vi "Esophogeal_HRME_Main.vi"() -> ()   [LabVIEW 2021]
uses:
  typeDefs/Esophogeal_Software_States.ctl
  <vilib>/DAQmx/read.llb/DAQmx Read (Digital 1D Bool NChan 1Samp 1Line).vi
  <extravilib>/ChannelInstances/High Speed Stream-str/_Read For Replicate.vi
  <extravilib>/ChannelInstances/High Speed Stream-a[.,.](u8)/_Read For Replicate.vi
  <vilib>/DAQmx/create/channels.llb/DAQmx Create Channel (DI-Digital Input).vi
  <vilib>/DAQmx/miscellaneous.llb/DAQmx Fill In Error Info.vi
  <extravilib>/ChannelInstances/High Speed Stream-str/Instantiate.vi
  <extravilib>/ChannelInstances/High Speed Stream-a[.,.](u8)/Instantiate.vi
  <extravilib>/ChannelInstances/High Speed Stream-str/)Channel.vi
  <extravilib>/ChannelInstances/High Speed Stream-str/Abort Signal/Init Signal.vi
  <extravilib>/ChannelInstances/High Speed Stream-a[.,.](u8)/)Channel.vi
  <extravilib>/ChannelInstances/High Speed Stream-a[.,.](u8)/Abort Signal/Init Signal.vi
  <vilib>/vision/driver/NI_Vision_Acquisition_Software.lvlib
  <resource>/objmgr/imaqdx.rc
  <extravilib>/ChannelInstances/High Speed Stream-a[.,.](u8).lvlib
  <extravilib>/ChannelInstances/High Speed Stream-str.lvlib
  <vilib>/vision/NI_Vision_Development_Module.lvlib
panel:
  out "Pause Status":bool
  in  "Tab Control":enum32{"Main Page", "Image Session Info"}(tab)
  in  "MTN Threshold:":enum16{"24.0", "15.9"}(ring)
  out "Image Analysis Meter":dbl(slide) scale=0.0..100.0
  in  "Calibrate":bool
  out "Saved Imaged Number":i32=1 caption="Number of Images Saved"
  out "Image Save Notification":string
  in  "Auto Gain":bool=TRUE
  in  "Auto Exposure":bool=TRUE
  in  "Save Button":bool
  out "Recording":bool
  in  "Play Button":bool
  in  "Close Program":bool
  in  "Pause Button":bool
  in  "HRME Gain":dbl(slide)=18.0 scale=0.0..30.0
  in  "HRME Exposure":dbl(slide)=7000.0 scale=100.0..80000.0
  out "HRME Image":T1(plugin-control)
  out "HRME Path":path
  out "HRME Scores":path
  out "Representative Images":path
  out "error out":errorcluster
  out "Patient Folder":path
  in  "Command File Location":path=path "C:/Users/EsophaHRME_Dell2/Documents/GitHub/Esophageal_HRME_Software/EsophagealDeployment/Multi_Task_Network/CommandFiles/LabVIEW/cmds.json"
  in  "Python Module Path":path=path "C:/Users/EsophaHRME_Dell2/Documents/GitHub/Esophageal_HRME_Software/EsophagealDeployment/Multi_Task_Network/mainv6.py"
  out "Log File Out":refnum<file>
  out "Anal HRME States":T2
  out "Timestamp":string
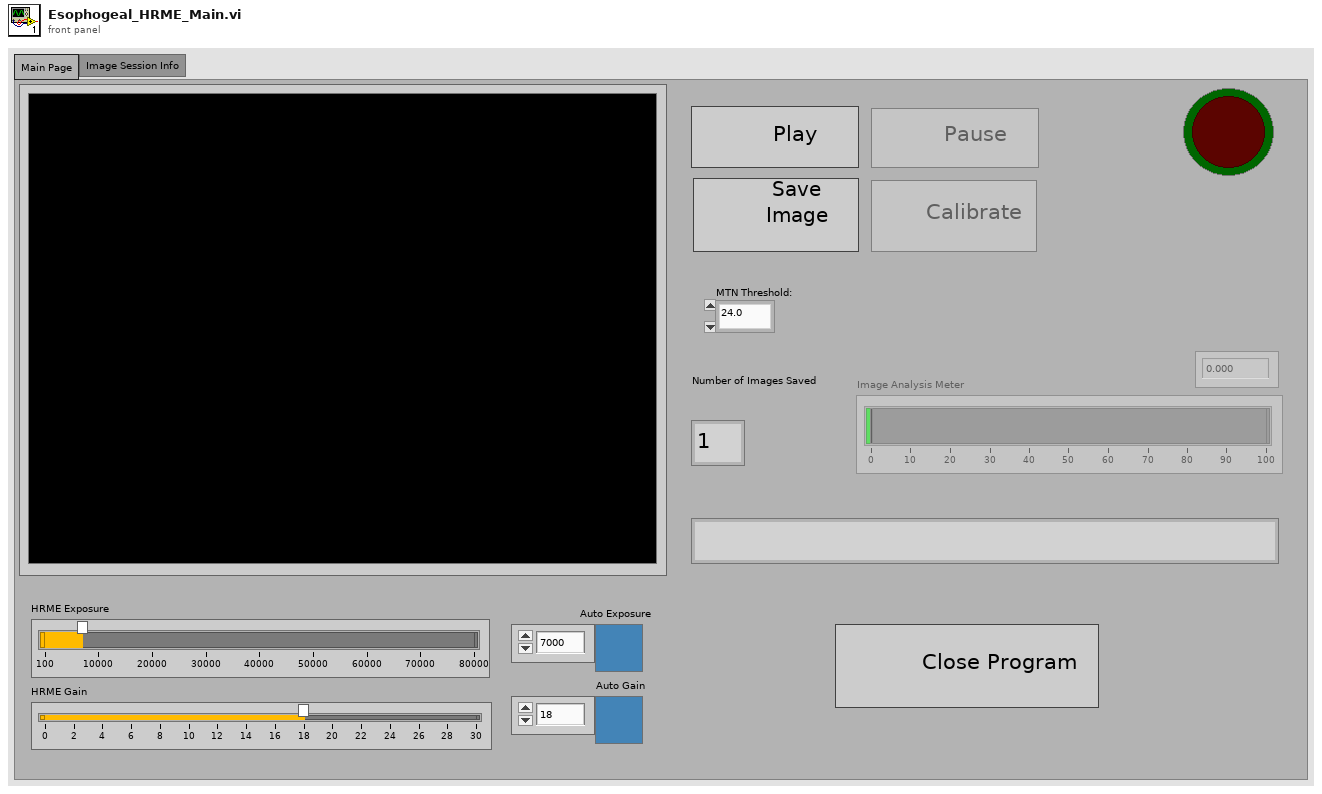
[diagram p1: front panel]
types:
  T1 = typedef "IMAQ Image.ctl" = refnum<image>
  T2 = typedef "Esophogeal_Software_States.ctl" = enum16{"Initialize", "Image Prep Screen", "Imaging", "Image Pause Screen", "Exit"}
  T3 = enum8{"Enabled", "Disabled", "Disabled and Grayed Out"}
  T4 = enum16{"open", "replace", "create", "open or create", "replace or create", "replace or create with confirmation"}
  T5 = cluster{"Source":string, "Destination":string, "CMD":string, "Time":string}
  T6 = typedef "IMAQdx.ctl" = refnum<k21>
  T7 = typedef "Image Type" = u32
  T8 = typedef "ROI Descriptor" = cluster{"Global Rectangle":i32[], "Contours":cluster{"ID":enum32{"External", "Internal"}, "Type":u32, "Coordinates":i32[]}[]}
  T9 = typedef "High Speed Stream-str.lvlib/)Channel.ctl" = refnum<queue>
  T10 = typedef "High Speed Stream-a[.,.](u8).lvlib/)Channel.ctl" = refnum<queue>
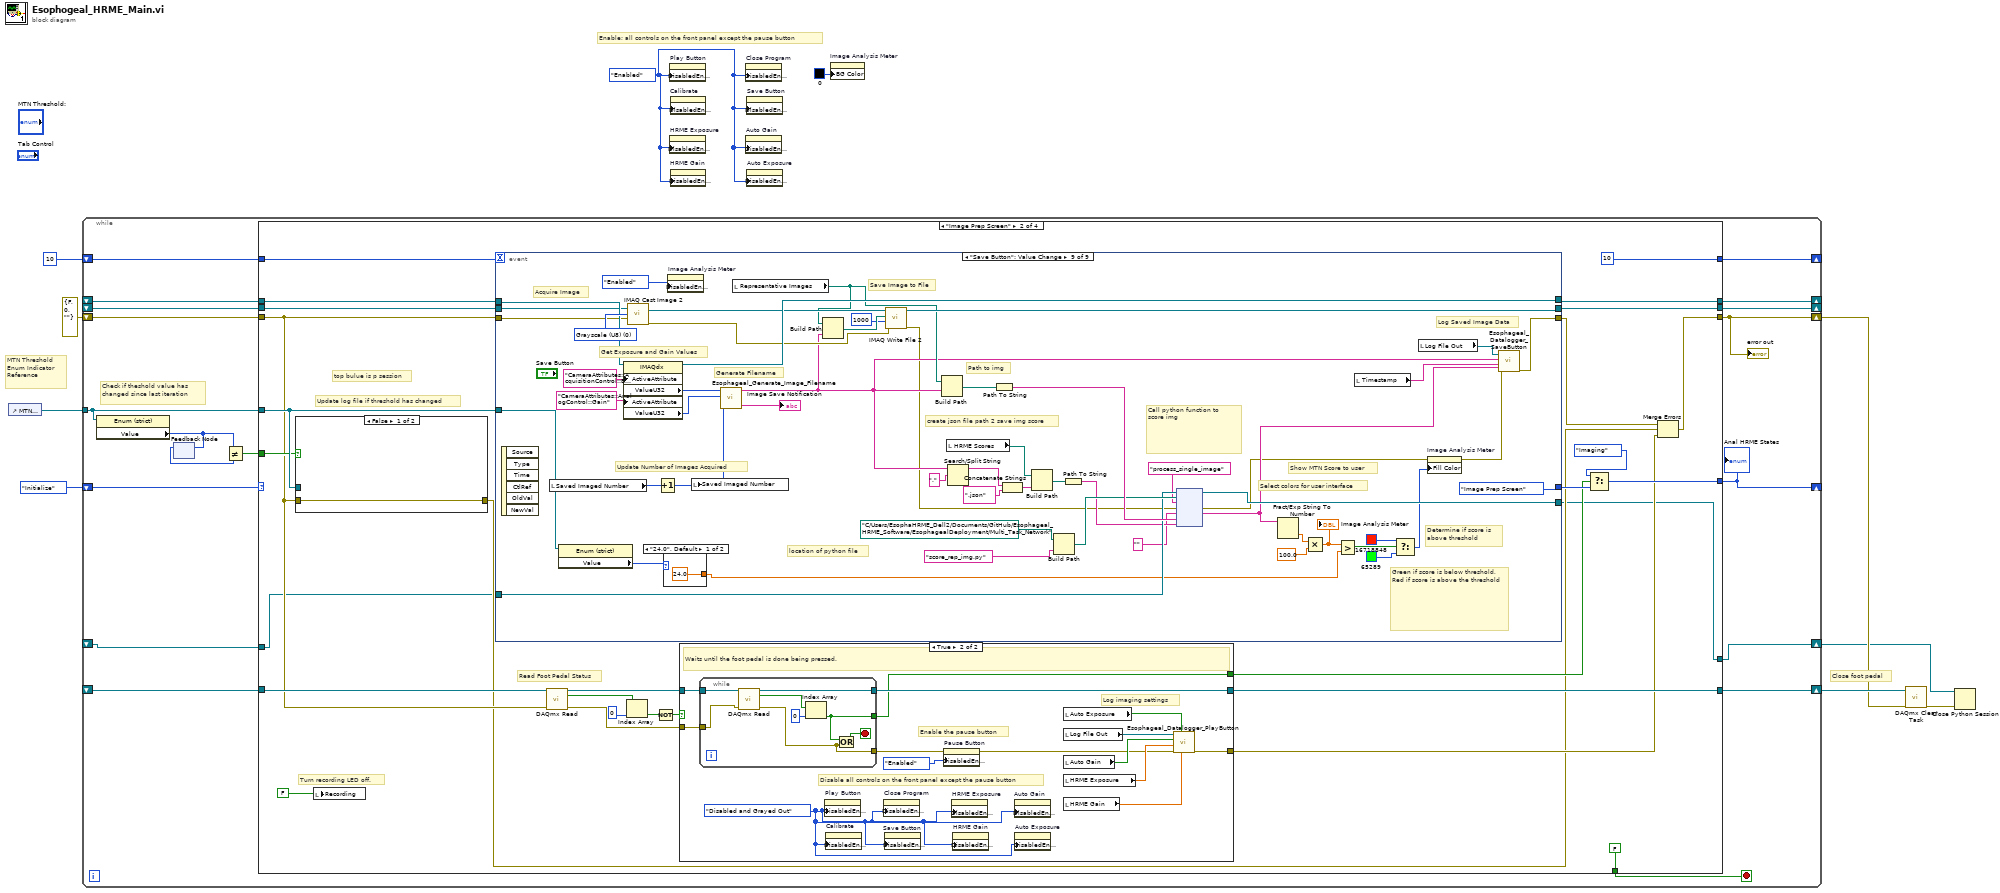
[diagram p0: block diagram]
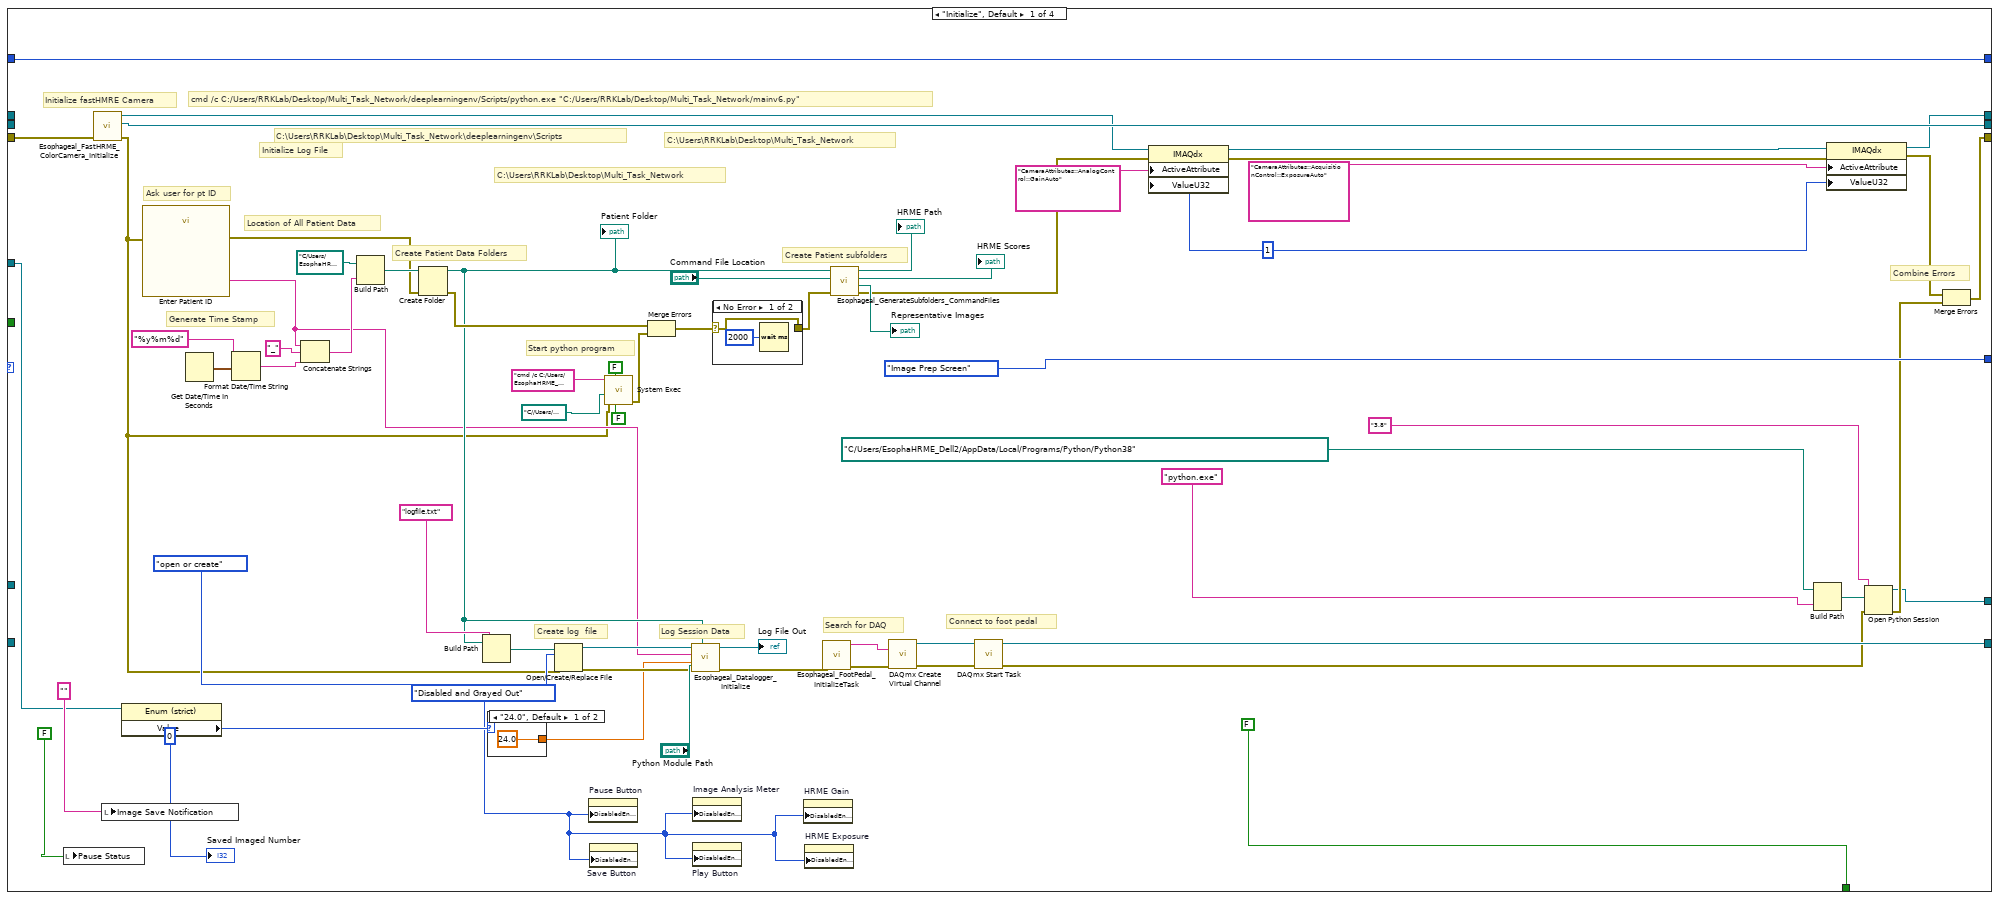
[diagram p2: hidden frame]
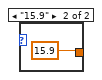
[diagram p3: hidden frame]
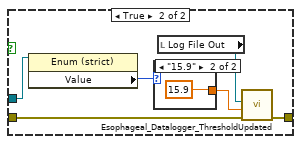
[diagram p5: hidden frame]
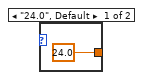
[diagram p6: hidden frame]
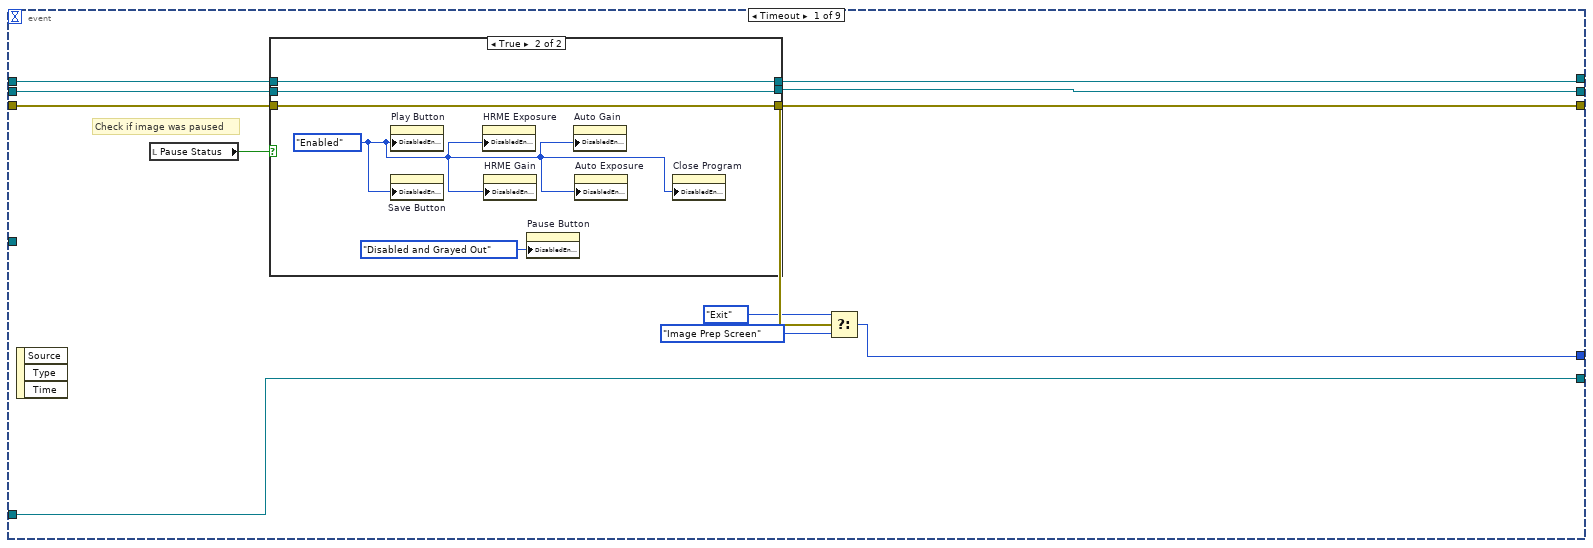
[diagram p8: hidden frame]
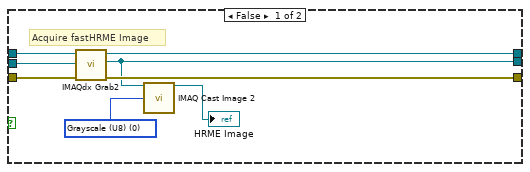
[diagram p9: hidden frame]
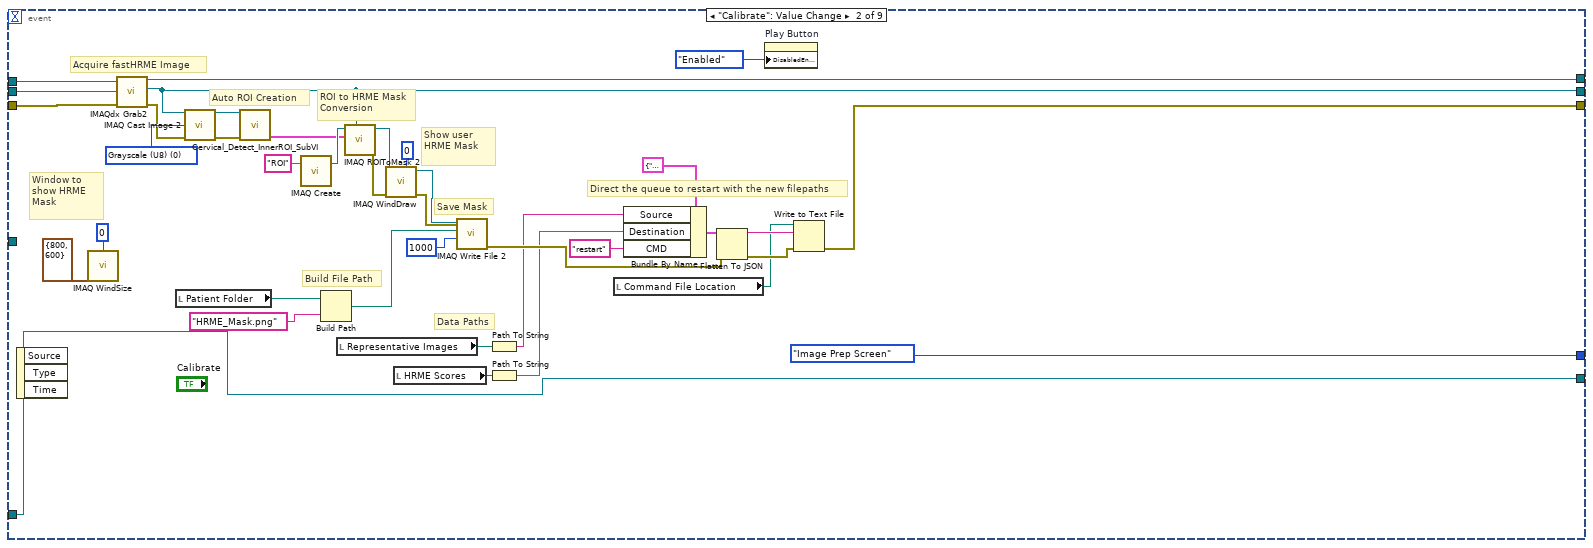
[diagram p10: hidden frame]
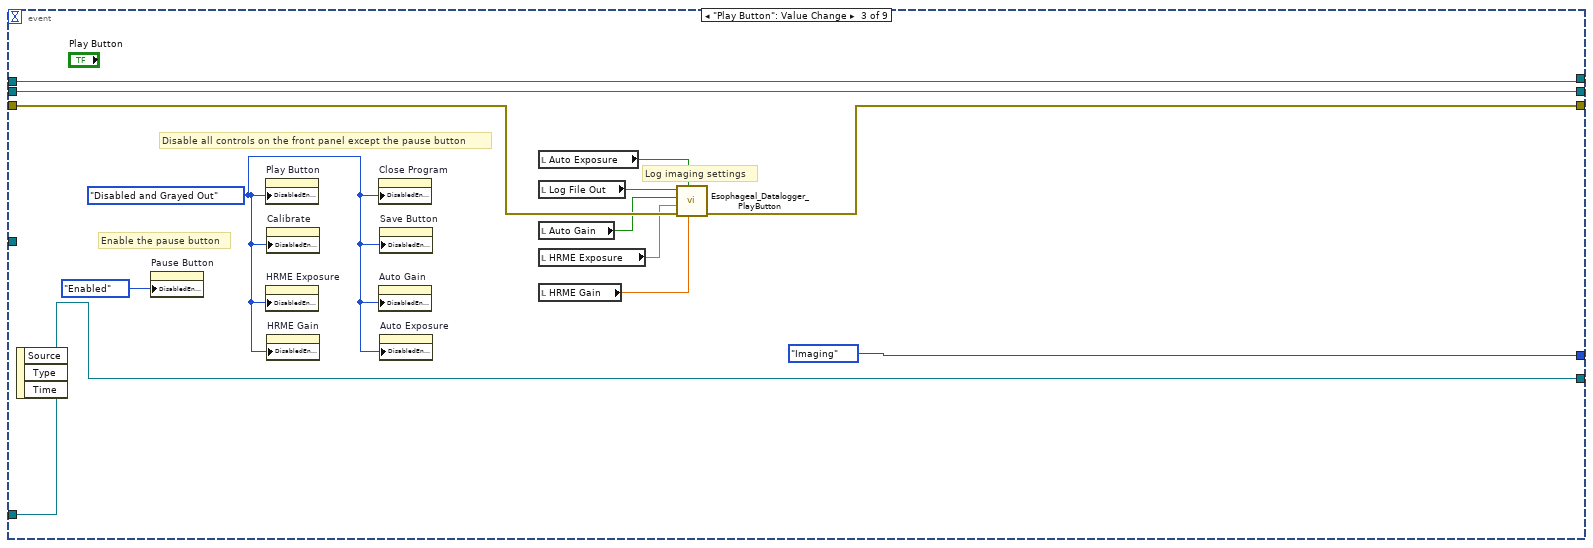
[diagram p11: hidden frame]
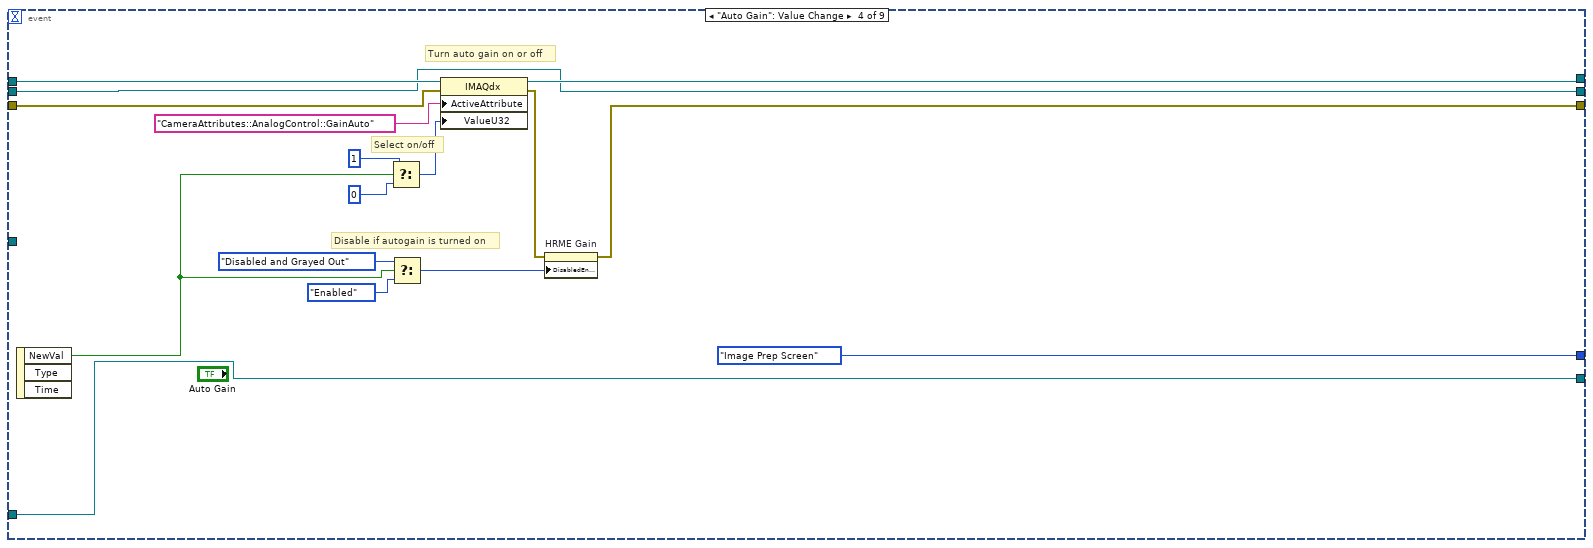
[diagram p12: hidden frame]
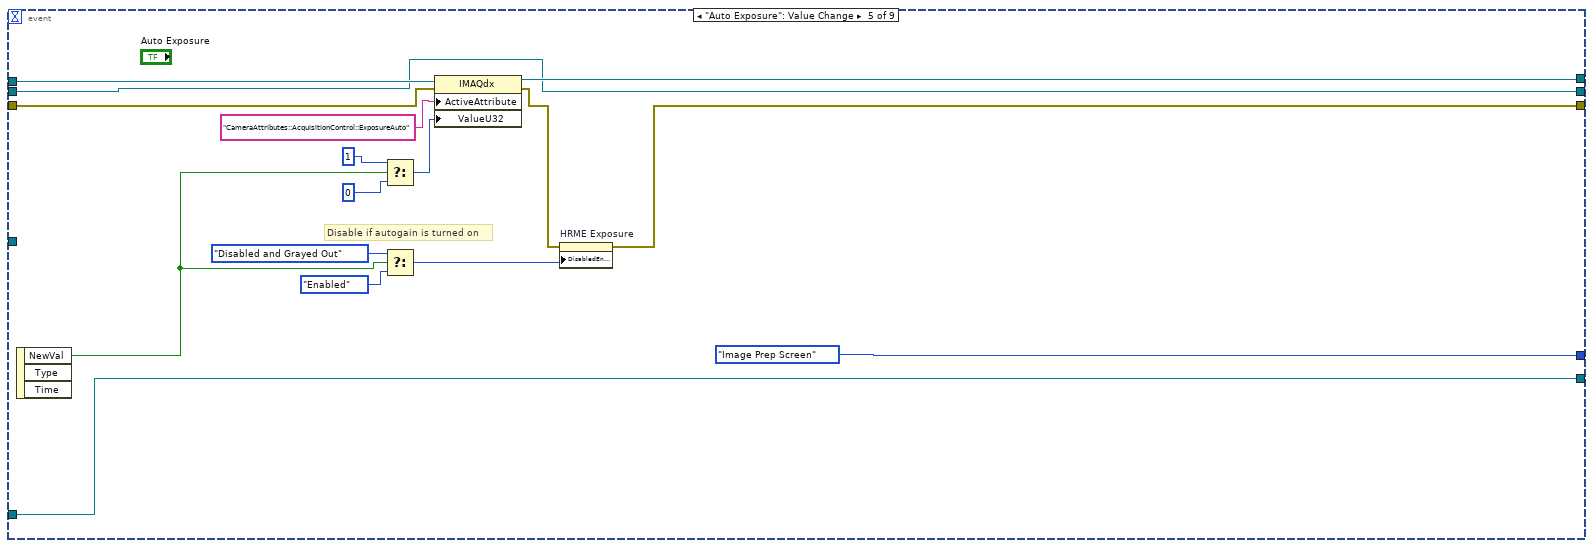
[diagram p13: hidden frame]
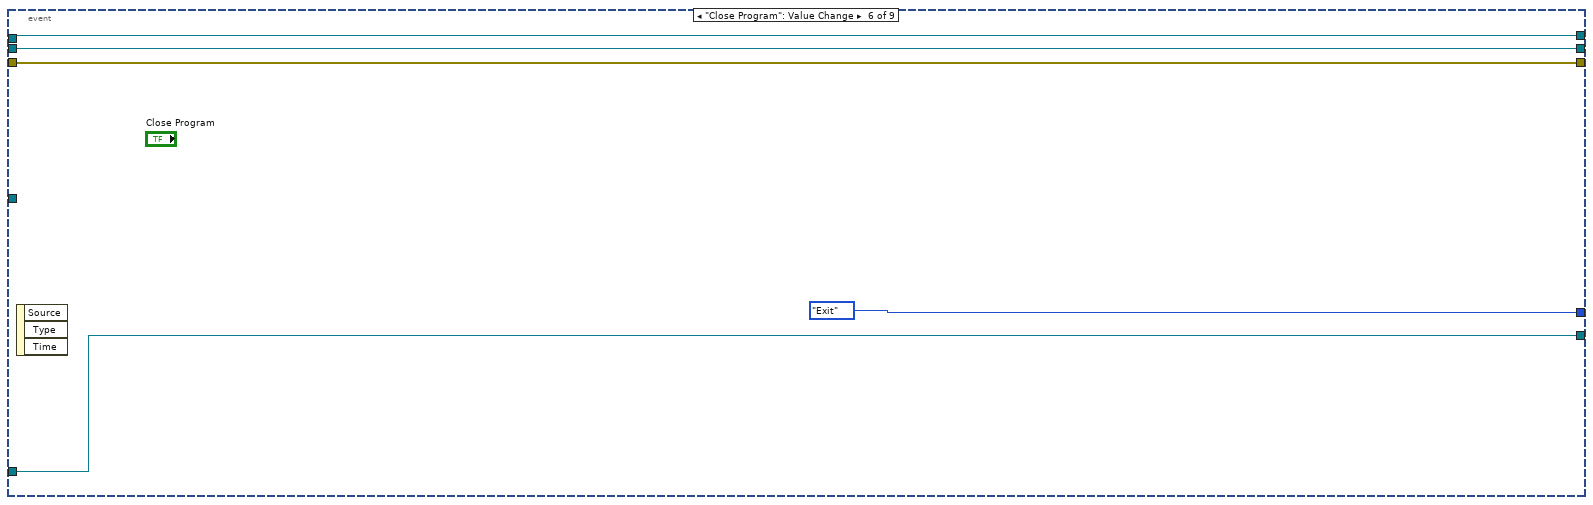
[diagram p14: hidden frame]
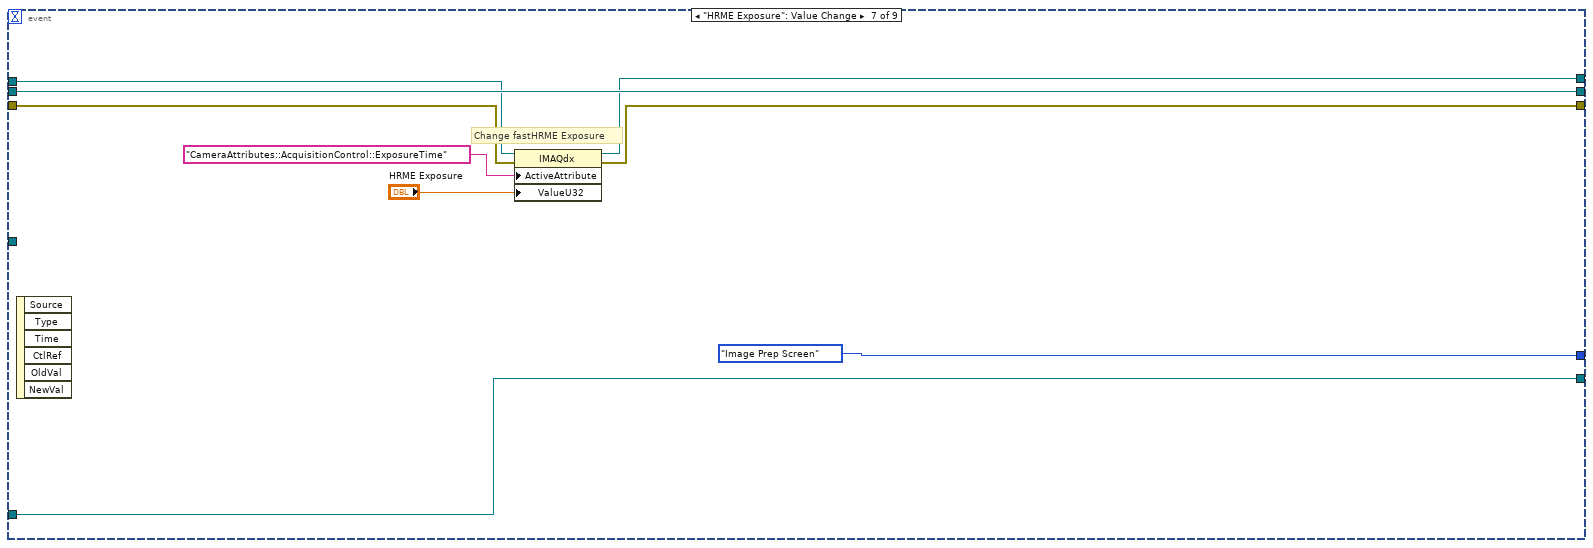
[diagram p15: hidden frame]
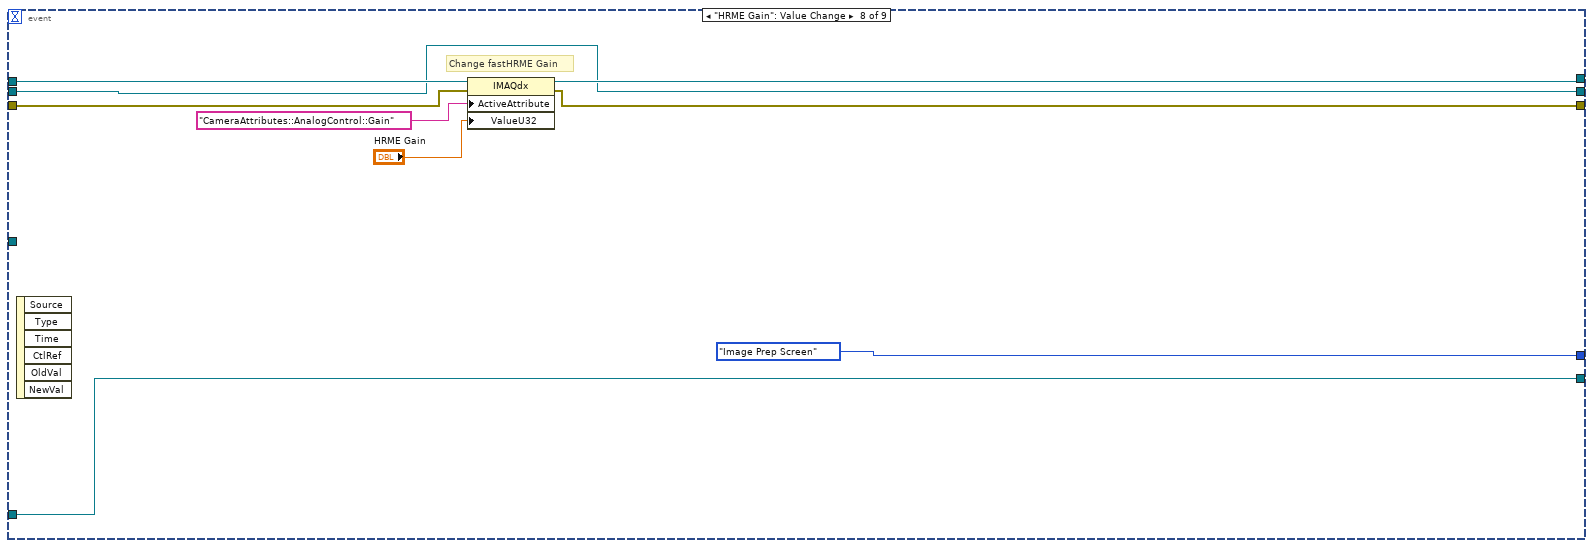
[diagram p16: hidden frame]
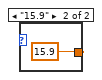
[diagram p17: hidden frame]
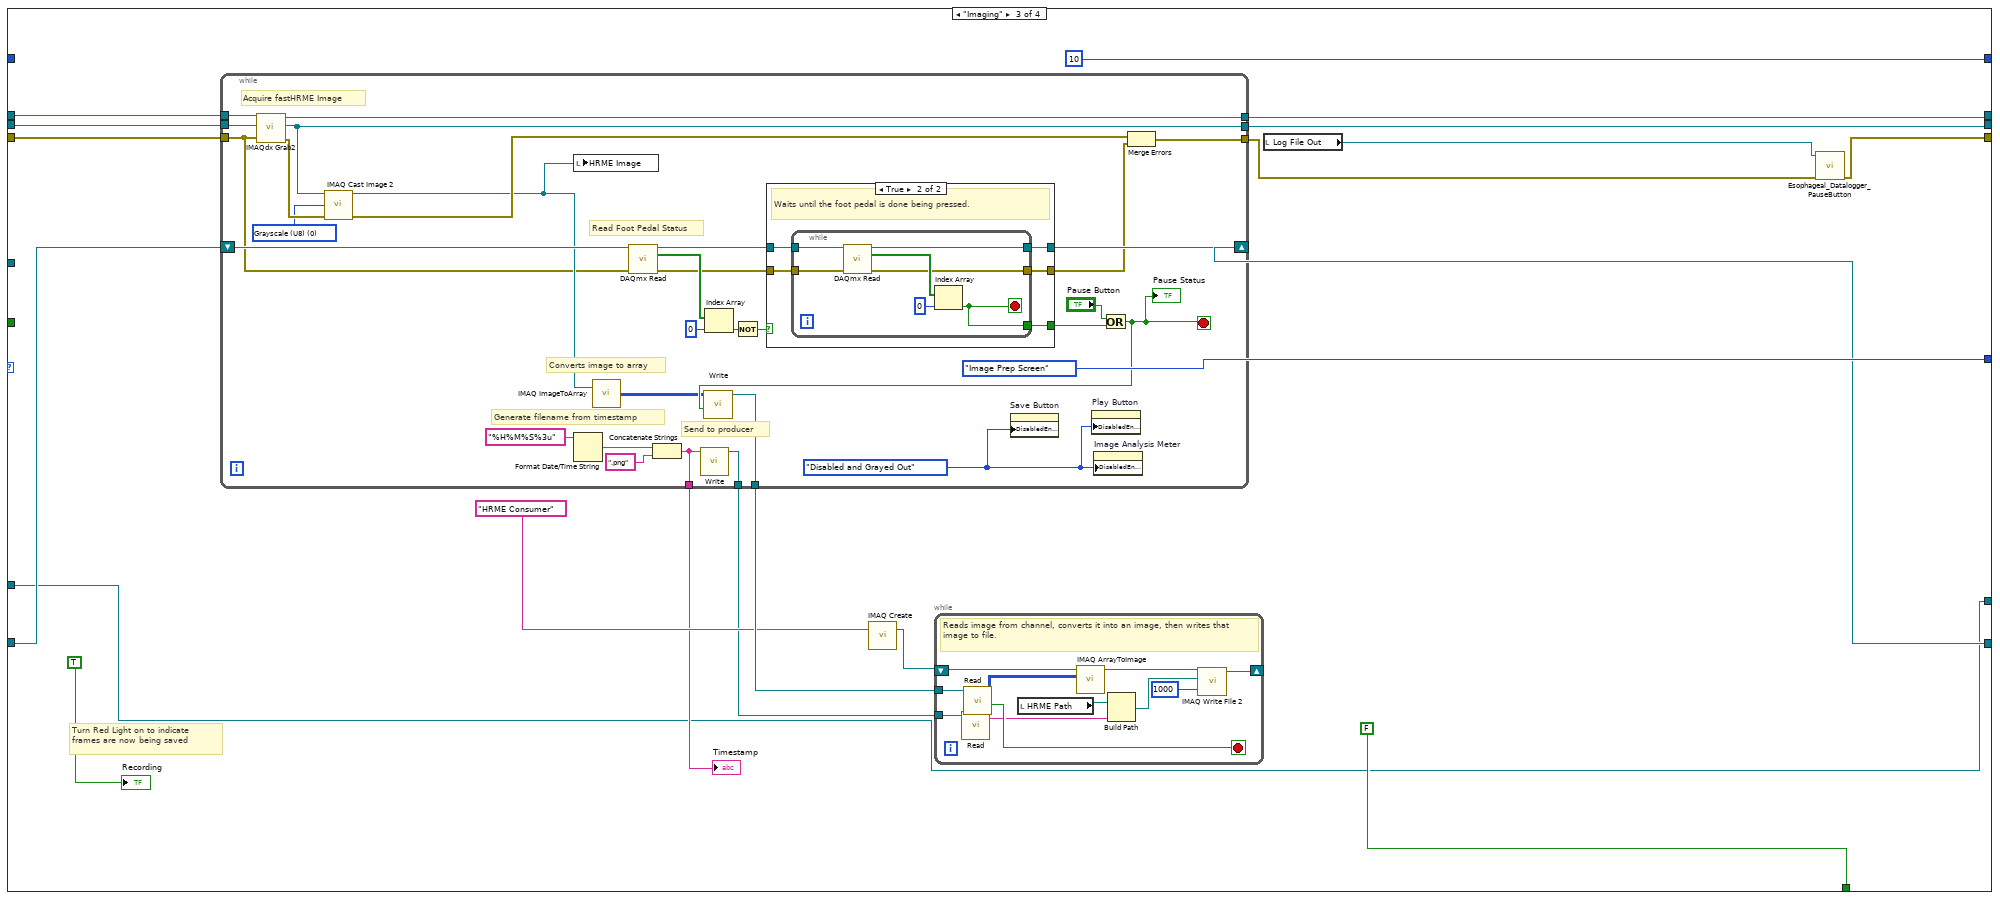
[diagram p18: hidden frame]
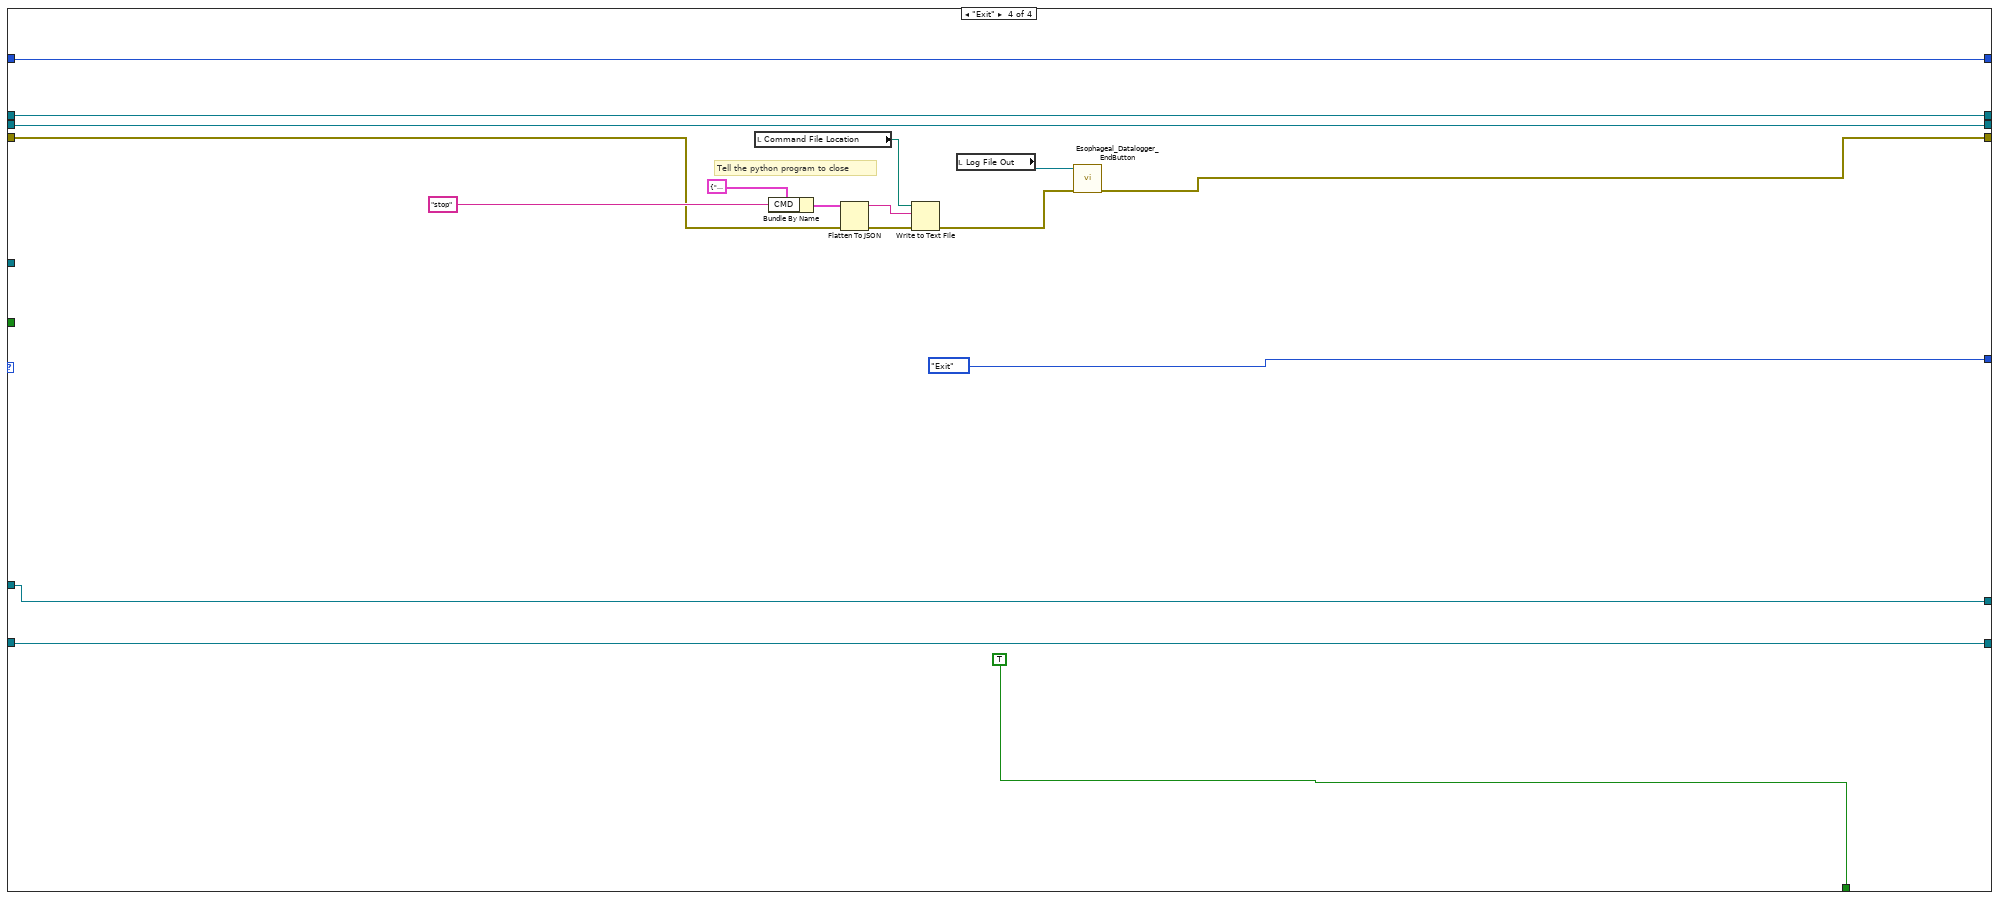
[diagram p20: hidden frame]
diagram:
  w5 = T3."Enabled" ("Disabled")
  # "MTN Threshold Enum Indicator Reference"
  # "Enable; all controls on the front panel except the pause button"
  # "Close foot pedal"
  n1 = control-ref of="MTN Threshold:"() -> (w3:refnum<vi>)
  n2 = while {
    shift-right: [w28] -> _
    shift-left: _ -> [w24]
    shift-right: [w27] -> _
    shift-left: _ -> [w23]
    shift-right: [w26] -> _
    shift-left: Esophogeal_Software_States."Initialize" ("Anal HRME States") -> [w29]
    shift-right: [w17] -> w8
    shift-left: errorcluster {"status"=FALSE, "code"=0, "source"=""} ("error IO") -> [w25]
    shift-right: [w20] -> w9
    shift-left: _ -> [w21]
    shift-right: [w18] -> _
    shift-left: 10 -> [w19]
    tunnel: w3 -> [w16]
    shift-right: [w12] -> w1
    shift-left: _ -> [w11]
    stop <- w22 stop-if-true
    # "Check if theshold value has changed since last iteration"
    n3 = property class="Enum (strict)"(reference=w16) -> ("Value"=w15:enum16{"24.0", "15.9"})  [unwired: 1 in, 2 out]
    n4 = feedback-in #1(w15) -> ()
    n5 = feedback #1() -> (w14:enum16{"24.0", "15.9"})  [unwired: 1 in]
    n6 = Not Equal?(x=w15, y=w14) -> (x != y?=w13:bool)
    n7 = case shown="\"Image Prep Screen\"" w29 {
      tunnel: [w41 w126 w364 w440] -> w28
      tunnel: [w94 w125 w363 w439] -> w27
      tunnel: [Esophogeal_Software_States."Image Prep Screen" ("Anal HRME States") w122 Esophogeal_Software_States."Image Prep Screen" ("Anal HRME States") Esophogeal_Software_States."Exit" ("Anal HRME States")] -> w26
      tunnel: w25 -> [w92 w105 w362 w429]
      tunnel: w24 -> [_ w128 w366 w440]
      tunnel: w23 -> [_ w127 w365 w439]
      tunnel: [FALSE FALSE FALSE TRUE] -> w22
      tunnel: [w38 w108 w351 w426] -> w17
      tunnel: w21 -> [_ w119 w361 w437]
      tunnel: [w88 w114 w358 w437] -> w20
      tunnel: w19 -> [w87 w112 _ w436]
      tunnel: [w87 10 10 w436] -> w18
      tunnel: w16 -> [w50 w107 _ _]
      tunnel: w13 -> [_ w106 _ _]
      tunnel: [w30 w101 w349 w425] -> w12
      tunnel: w11 -> [_ w102 w349 w425]
      frame "Initialize", Default {
        w37 = 1
        w47 = T3."Disabled and Grayed Out" ("Disabled")
        # "C:\\Users\\RRKLab\\Desktop\\Multi_Task_Network"
        # "C:\\Users\\RRKLab\\Desktop\\Multi_Task_Network"
        # "C:\\Users\\RRKLab\\Desktop\\Multi_Task_Network\\deeplearningenv\\Scripts"
        # "cmd /c C:/Users/RRKLab/Desktop/Multi_Task_Network/deeplearningenv/Scripts/python.exe \"C:/Users/RRKLab/Desktop/Multi_Task_Network/mainv6.py\""
        # "Create log  file"
        # "Log Session Data"
        # "Initialize Log File"
        # "Create Patient subfolders"
        # "Search for DAQ"
        # "Start python program"
        # "Location of All Patient Data"
        # "Combine Errors"
        # "Create Patient Data Folders"
        # "Generate Time Stamp"
        # "Ask user for pt ID"
        # "Connect to foot pedal"
        # "Initialize fastHMRE Camera"
        n8 = local write "Pause Status"(FALSE ("Pause Status")) -> ()
        n9 = call "Esophageal_FastHRME_ColorCamera_Initialize.vi"("error in (no error)"=w92) -> ("error out"=w51:errorcluster, "HRME Image Reference"=w94:T1, "OMS Camera Reference Out"=w42:T6)  [unwired: 8 in]
        n10 = local write "Image Save Notification"("" ("Image Save Notification")) -> ()
        n11 = property class="Enum (strict)"(reference=w50) -> ("Value"=w49:enum16{"24.0", "15.9"})  [unwired: 1 in, 2 out]
        n12 = call "Enter Patient ID"("error in (no error)"=w51) -> ("Patient ID"=w52:string, "error out"=w78:errorcluster)  [unwired: 16 in, 1 out]
        n13 = Get Date/Time In Seconds() -> (seconds since 1Jan1904=w84:timestamp)
        n14 = Format Date/Time String(time format string (%c)="%y%m%d", seconds (now)=w84) -> (date/time string=w81:string)  [unwired: 1 in]
        n15 = Concatenate Strings(w52, "_" ("string"), w81) -> (w80:string)
        n16 = Build Path(base path=path "C:/Users/EsophaHRME_Dell2/Desktop/PatientData", name or relative path=w80) -> (appended path=w79:path)
        n17 = Create Folder(path (use dialog)=w79, error in=w78) -> (created path=w53:path, error out=w67:errorcluster)  [unwired: 1 in, 1 out]
        "Patient Folder" <- w53
        n18 = Build Path(base path=w53, name or relative path="logfile.txt") -> (appended path=w55:path)
        n19 = case shown="\"24.0\", Default" w49 {
          tunnel: [24.0 15.9] -> w48
          frame "24.0", Default {
          }
          frame "15.9" {
          }
        }
        n20 = Open/Create/Replace File(file path (use dialog)=w55, error in=w51, operation (0:open)=T4."open or create") -> (refnum out=w58:refnum<file>, error out=w59:errorcluster)  [unwired: 3 in, 1 out]
        n21 = property on="Pause Button" class="Bool"("DisabledEnum"=w47) -> ()  [unwired: 2 in, 2 out]
        n22 = property on="Save Button" class="Bool"("DisabledEnum"=w47) -> ()  [unwired: 2 in, 2 out]
        n23 = call <vilib>:"System Exec.vi"("run minimized? (F)"=FALSE, "wait until completion? (T)"=FALSE, "error in (no error)"=w51, "working directory"=path "C://Users/EsophaHRME_Dell2/Documents/GitHub/Esophageal_HRME_Software/EsophagealDeployment/Multi_Task_Network", "command line"="cmd /c C:/Users/EsophaHRME_Dell2/anaconda3/envs/esophaenv/python.exe \"C:/Users/EsophaHRME_Dell2/Documents/GitHub/Esophageal_HRME_Software/EsophagealDeployment/Multi_Task_Network/mainv6.py\"") -> ("error out"=w66:errorcluster)  [unwired: 3 in, 3 out]
        n24 = Merge Errors(w67, w66) -> (w68:errorcluster)
        n25 = call "Esophageal_Datalogger_Initialize.vi"("Python Module Path"="Python Module Path", "Data File Path"=w53, "error in (no error)"=w59, "MTN Threshold"=w48, "Patient ID"=w52, "Log File In"=w58) -> ("error out"=w54:errorcluster, "Log File Out"=→"Log File Out":refnum<file>)  [unwired: 4 in]
        n26 = property on="Image Analysis Meter" class="Slide (strict)"("DisabledEnum"=w47) -> ()  [unwired: 2 in, 2 out]
        n27 = property on="Play Button" class="Bool"("DisabledEnum"=w47) -> ()  [unwired: 2 in, 2 out]
        n28 = case shown="No Error" w68 {
          selector: w68 -> [w97 w99]
          tunnel: [w97 w99] -> w72
          frame No Error {
            n29 = Wait (ms)(milliseconds to wait=u32 2000) -> ()  [unwired: 1 out]
          }
          frame Error {
          }
        }
        n30 = property on="HRME Gain" class="Slide (strict)"("DisabledEnum"=w47) -> ()  [unwired: 2 in, 2 out]
        n31 = property on="HRME Exposure" class="Slide (strict)"("DisabledEnum"=w47) -> ()  [unwired: 2 in, 2 out]
        n32 = call "Esophageal_FootPedal_InitializeTask.vi"("error in (no error)"=w54) -> ("error out"=w64:errorcluster, "Task Command"=w63:string)  [unwired: 9 in]
        n33 = call "Esophageal_GenerateSubfolders_CommandFiles.vi"("error in"=w72, "Command File Location"="Command File Location", "Patient Data Folder"=w53) -> ("error out"=w45:errorcluster, "Rep Image Path"=→"Representative Images":path, "HRME Scores"=→"HRME Scores":path, "HRME Path"=→"HRME Path":path)  [unwired: 5 in]
        n34 = call-poly <vilib>:"DAQmx Create Virtual Channel.vi"("lines"=w63, "error in"=w64) -> ("task out"=w89:refnum<k21>, "error out"=w90:errorcluster)  [unwired: 12 in]
        n35 = call <vilib>:"DAQmx Start Task.vi"("task/channels in"=w89, "error in"=w90) -> ("task out"=w88:refnum<k21>, "error out"=w33:errorcluster)  [unwired: 12 in]
        n36 = property class="IMAQdx"(reference=w42, error in=w45, "ActiveAttribute"="CameraAttributes::AnalogControl::GainAuto", "ValueU32"=w37) -> (reference out=w43:T6, error out=w40:errorcluster)
        n37 = Build Path(base path=path "C:/Users/EsophaHRME_Dell2/AppData/Local/Programs/Python/Python38", name or relative path="python.exe") -> (appended path=w35:path)
        n38 = property class="IMAQdx"(reference=w43, error in=w40, "ActiveAttribute"="CameraAttributes::AcquisitionControl::ExposureAuto", "ValueU32"=w37) -> (reference out=w41:T6, error out=w39:errorcluster)
        n39 = Open Python Session(python version="3.8", python path=w35, 3:w33) -> (session out=w30:refnum<k35>, error out=w32:errorcluster)
        n40 = Merge Errors(w39, w32) -> (w38:errorcluster)
        "Saved Imaged Number" <- 0
      }
      frame "Image Prep Screen" {
        # "top bulue is p session"
        # "Update log file if threshold has changed"
        # "Turn recording LED off."
        # "Read Foot Pedal Status"
        n41 = case shown="False" w106 {
          tunnel: w107 -> [_ w135]
          tunnel: w105 -> [w129 w131]
          tunnel: [w129 w130] -> w103
          frame False {
          }
          frame True {
            n42 = property class="Enum (strict)"(reference=w135) -> ("Value"=w134:enum16{"24.0", "15.9"})  [unwired: 1 in, 2 out]
            n43 = case shown="\"15.9\"" w134 {
              tunnel: [24.0 15.9] -> w133
              frame "24.0", Default {
              }
              frame "15.9" {
              }
            }
            n44 = local read "Log File Out"() -> (w132:refnum<file>)
            n45 = call "Esophageal_Datalogger_ThresholdUpdated.vi"("error in"=w131, "MTN Threshold"=w133, "Log File In"=w132) -> ("error out"=w130:errorcluster)  [unwired: 7 in, 1 out]
          }
        }
        n46 = local write "Recording"(FALSE ("Recording")) -> ()
        n47 = event shown="[8] \"Save Button\": Value Change" {
          selector: _ -> [_ _ _ _ _ _ _ _ _]
          dyn-events: _ -> [_ _ _ _ _ _ _ _ _]
          timeout: w112 -> [_ _ _ _ _ _ _ _ _]
          tunnel: w128 -> [w173 w223 w236 w253 w266 w273 w281 w290 w330]
          tunnel: w127 -> [w171 w222 w235 w250 w263 w272 w282 w286 w329]
          tunnel: [w165 Esophogeal_Software_States."Image Prep Screen" ("Anal HRME States") Esophogeal_Software_States."Imaging" ("Anal HRME States") Esophogeal_Software_States."Image Prep Screen" ("Anal HRME States") Esophogeal_Software_States."Image Prep Screen" ("Anal HRME States") Esophogeal_Software_States."Exit" ("Anal HRME States") Esophogeal_Software_States."Image Prep Screen" ("Anal HRME States") Esophogeal_Software_States."Image Prep Screen" ("Anal HRME States") Esophogeal_Software_States."Image Prep Screen" ("Anal HRME States")] -> w121
          tunnel: [w172 w220 w236 w252 w265 w273 w280 w289 w341] -> w126
          tunnel: [w170 w198 w235 w250 w263 w272 w282 w286 w344] -> w125
          tunnel: w105 -> [w169 w221 w231 w251 w264 w271 w277 w287 w322]
          tunnel: [w166 w206 w230 w241 w259 w271 w276 w288 w328] -> w109
          tunnel: w107 -> [_ _ _ _ _ _ _ _ w323]
          tunnel: w102 -> [w163 w187 w225 w238 w254 w270 w275 w284 w308]
          tunnel: [w163 w187 w225 w238 w254 w270 w275 w284 w307] -> w101
          event Timeout {
            # "Check if image was paused"
            n48 = event-data() -> ()  [unwired: 1 in, 3 out]
            n49 = local read "Pause Status"() -> (w168:bool)
            n50 = case shown="True" w168 {
              tunnel: w173 -> [w181 w186]
              tunnel: [w180 w186] -> w172
              tunnel: w171 -> [w179 w185]
              tunnel: [w175 w185] -> w170
              tunnel: w169 -> [w178 w183]
              tunnel: [w177 w183] -> w166
              frame False {
                w174 = T7 0 items=["Grayscale (U8)", "Grayscale (I16)", "Grayscale (SGL)", "Complex (CSG)", "RGB (U32)", "HSL (U32)", "RGB (U64)", "Grayscale (U16)"] ("Image Type")
                # "Acquire fastHRME Image"
                n51 = call <vilib>:"IMAQdx Grab2.vi"("error in"=w178, "Image In"=w179, "Session In"=w181) -> ("error out"=w177:errorcluster, "Image Out"=w175:T1, "Session Out"=w180:T6)  [unwired: 5 in, 1 out]
                n52 = call "IMAQ Cast Image 2"("Image Src"=w175, "Image Type"=w174) -> ("Image Dst Out"=→"HRME Image":T1)  [unwired: 12 in, 1 out]
              }
              frame True {
                w182 = T3."Enabled" ("Disabled")
                n53 = property on="Play Button" class="Bool"("DisabledEnum"=w182) -> ()  [unwired: 2 in, 2 out]
                n54 = property on="Save Button" class="Bool"("DisabledEnum"=w182) -> ()  [unwired: 2 in, 2 out]
                n55 = property on="HRME Exposure" class="Slide (strict)"("DisabledEnum"=w182) -> ()  [unwired: 2 in, 2 out]
                n56 = property on="HRME Gain" class="Slide (strict)"("DisabledEnum"=w182) -> ()  [unwired: 2 in, 2 out]
                n57 = property on="Pause Button" class="Bool"("DisabledEnum"=T3."Disabled and Grayed Out" ("Disabled")) -> ()  [unwired: 2 in, 2 out]
                n58 = property on="Auto Gain" class="Bool (strict)"("DisabledEnum"=w182) -> ()  [unwired: 2 in, 2 out]
                n59 = property on="Auto Exposure" class="Bool (strict)"("DisabledEnum"=w182) -> ()  [unwired: 2 in, 2 out]
                n60 = property on="Close Program" class="Bool"("DisabledEnum"=w182) -> ()  [unwired: 2 in, 2 out]
              }
            }
            n61 = Select(t=Esophogeal_Software_States."Exit" ("Anal HRME States"), s=w166, f=Esophogeal_Software_States."Image Prep Screen" ("Anal HRME States")) -> (s? t:f=w165:T2)
          }
          event "Calibrate": Value Change {
            w224 = T7 0 items=["Grayscale (U8)", "Grayscale (I16)", "Grayscale (SGL)", "Complex (CSG)", "RGB (U32)", "HSL (U32)", "RGB (U64)", "Grayscale (U16)"] ("Image Type")
            # "ROI to HRME Mask Conversion"
            # "Show user HRME Mask"
            # "Window to show HRME Mask"
            # "Auto ROI Creation"
            # "Data Paths"
            # "Direct the queue to restart with the new filepaths"
            # "Build File Path"
            # "Save Mask"
            # "Acquire fastHRME Image"
            n62 = event-data() -> ()  [unwired: 1 in, 3 out]
            n63 = call "IMAQ WindSize"("Width & Height"=cluster{"Width":i32, "Height":i32} {"Width"=800, "Height"=600}, "Window Number"=0) -> ()  [unwired: 4 in, 3 out]
            n64 = call <vilib>:"IMAQdx Grab2.vi"("error in"=w221, "Image In"=w222, "Session In"=w223) -> ("error out"=w212:errorcluster, "Image Out"=w198:T1, "Session Out"=w220:T6)  [unwired: 5 in, 1 out]
            n65 = local read "Patient Folder"() -> (w218:path)
            n66 = call "IMAQ Cast Image 2"("Image Src"=w198, "Image Type"=w224, "error in (no error)"=w212) -> ("Image Dst Out"=w190:T1, "error out"=w191:errorcluster)  [unwired: 11 in]
            n67 = call "Cervical_Detect_InnerROI_SubVI.vi"("error in"=w191, "Raw Image"=w190) -> ("ROI Descriptor"=w189:T8)  [unwired: 6 in, 3 out]
            n68 = call "IMAQ Create"("Image Name"="ROI") -> ("New Image"=w213:T1)  [unwired: 4 in, 1 out]
            n69 = Build Path(base path=w218, name or relative path="HRME_Mask.png") -> (appended path=w216:path)
            n70 = local read "Representative Images"() -> (w203:path)
            n71 = call "IMAQ ROIToMask 2"("Image Model"=w198, "ROI Descriptor"=w189, "Image"=w213) -> ("error out"=w193:errorcluster, "Image Out"=w194:T1)  [unwired: 6 in, 1 out]
            n72 = call "IMAQ WindDraw"("Window Number (0...15)"=0 ("Window Number"), "error in (no error)"=w193, "Image"=w194) -> ("error out"=w192:errorcluster, "Image Out (duplicate)"=w188:T1)  [unwired: 7 in]
            n73 = local read "HRME Scores"() -> (w202:path)
            n74 = call-poly "IMAQ Write File 2"("error in (no error)"=w192, "Image Quality"=u32 1000, "File Path"=w216, "Image"=w188) -> ("error out"=w208:errorcluster)  [unwired: 6 in, 1 out]
            n75 = Path To String(path=w203) -> (string=w201:string)
            n76 = Path To String(path=w202) -> (string=w200:string)
            n77 = local read "Command File Location"() -> (w204:path)
            n78 = Bundle By Name(cluster=T5 {"Source"="", "Destination"="", "CMD"="newfolders", "Time"="time"} ("Output JSON File"), "Source"=w201, "Destination"=w200, "CMD"="restart") -> (w210:T5)
            n79 = Flatten To JSON(anything=w210, error in (no error)=w208) -> (JSON string=w211:string, 11:w207:errorcluster)  [unwired: 1 in]
            n80 = property on="Play Button" class="Bool"("DisabledEnum"=T3."Enabled" ("Disabled")) -> ()  [unwired: 2 in, 2 out]
            n81 = Write to Text File(file (use dialog)=w204, text=w211, error in=w207) -> (error out=w206:errorcluster)  [unwired: 1 in, 2 out]
          }
          event "Play Button": Value Change {
            w233 = T3."Disabled and Grayed Out" ("Disabled")
            # "Log imaging settings"
            # "Enable the pause button"
            # "Disable all controls on the front panel except the pause button"
            n82 = event-data() -> ()  [unwired: 1 in, 3 out]
            n83 = property on="Pause Button" class="Bool"("DisabledEnum"=T3."Enabled" ("Disabled")) -> ()  [unwired: 2 in, 2 out]
            n84 = property on="Play Button" class="Bool"("DisabledEnum"=w233) -> ()  [unwired: 2 in, 2 out]
            n85 = property on="HRME Exposure" class="Slide (strict)"("DisabledEnum"=w233) -> ()  [unwired: 2 in, 2 out]
            n86 = property on="Calibrate" class="Bool"("DisabledEnum"=w233) -> ()  [unwired: 2 in, 2 out]
            n87 = property on="HRME Gain" class="Slide (strict)"("DisabledEnum"=w233) -> ()  [unwired: 2 in, 2 out]
            n88 = property on="Close Program" class="Bool"("DisabledEnum"=w233) -> ()  [unwired: 2 in, 2 out]
            n89 = property on="Auto Gain" class="Bool (strict)"("DisabledEnum"=w233) -> ()  [unwired: 2 in, 2 out]
            n90 = property on="Save Button" class="Bool"("DisabledEnum"=w233) -> ()  [unwired: 2 in, 2 out]
            n91 = property on="Auto Exposure" class="Bool (strict)"("DisabledEnum"=w233) -> ()  [unwired: 2 in, 2 out]
            n92 = local read "Auto Exposure"() -> (w229:bool)
            n93 = local read "Log File Out"() -> (w232:refnum<file>)
            n94 = local read "Auto Gain"() -> (w228:bool)
            n95 = local read "HRME Exposure"() -> (w227:dbl)
            n96 = local read "HRME Gain"() -> (w226:dbl)
            n97 = call "Esophageal_Datalogger_PlayButton.vi"("Gain Value"=w226, "Auto Exposure Status"=w229, "error in (no error)"=w231, "Exposure Value"=w227, "Auto Gain Status"=w228, "Log File In"=w232) -> ("error out"=w230:errorcluster)  [unwired: 4 in, 1 out]
          }
          event "Auto Gain": Value Change {
            # "Disable if autogain is turned on"
            # "Select on/off"
            # "Turn auto gain on or off"
            n98 = event-data() -> ("NewVal"=w244:bool)  [unwired: 1 in, 2 out]
            n99 = Select(t=u32 1 ("ValueU32"), s=w244, f=u32 0 ("ValueU32")) -> (s? t:f=w247:u32)
            n100 = Select(t=T3."Disabled and Grayed Out" ("Disabled"), s=w244, f=T3."Enabled" ("Disabled")) -> (s? t:f=w243:T3)
            n101 = property class="IMAQdx"(reference=w253, error in=w251, "ActiveAttribute"="CameraAttributes::AnalogControl::GainAuto", "ValueU32"=w247) -> (reference out=w252:T6, error out=w242:errorcluster)
            n102 = property on="HRME Gain" class="Slide (strict)"(error in=w242, "DisabledEnum"=w243) -> (error out=w241:errorcluster)  [unwired: 1 in, 1 out]
          }
          event "Auto Exposure": Value Change {
            # "Disable if autogain is turned on"
            n103 = event-data() -> ("NewVal"=w257:bool)  [unwired: 1 in, 2 out]
            n104 = Select(t=u32 1 ("ValueU32"), s=w257, f=u32 0 ("ValueU32")) -> (s? t:f=w269:u32)
            n105 = Select(t=T3."Disabled and Grayed Out" ("Disabled"), s=w257, f=T3."Enabled" ("Disabled")) -> (s? t:f=w258:T3)
            n106 = property class="IMAQdx"(reference=w266, error in=w264, "ActiveAttribute"="CameraAttributes::AcquisitionControl::ExposureAuto", "ValueU32"=w269) -> (reference out=w265:T6, error out=w260:errorcluster)
            n107 = property on="HRME Exposure" class="Slide (strict)"(error in=w260, "DisabledEnum"=w258) -> (error out=w259:errorcluster)  [unwired: 1 in, 1 out]
          }
          event "Close Program": Value Change {
            n108 = event-data() -> ()  [unwired: 1 in, 3 out]
          }
          event "HRME Exposure": Value Change {
            # "Change fastHRME Exposure"
            n109 = event-data() -> ()  [unwired: 1 in, 6 out]
            n110 = property class="IMAQdx"(reference=w281, error in=w277, "ActiveAttribute"="CameraAttributes::AcquisitionControl::ExposureTime", "ValueU32"="HRME Exposure") -> (reference out=w280:T6, error out=w276:errorcluster)
          }
          event "HRME Gain": Value Change {
            # "Change fastHRME Gain"
            n111 = event-data() -> ()  [unwired: 1 in, 6 out]
            n112 = property class="IMAQdx"(reference=w290, error in=w287, "ActiveAttribute"="CameraAttributes::AnalogControl::Gain", "ValueU32"="HRME Gain") -> (reference out=w289:T6, error out=w288:errorcluster)
          }
          event "Save Button": Value Change {
            w334 = T7 0 items=["Grayscale (U8)", "Grayscale (I16)", "Grayscale (SGL)", "Complex (CSG)", "RGB (U32)", "HSL (U32)", "RGB (U64)", "Grayscale (U16)"] ("Image Type")
            # "Path to img"
            # "Green if score is below threshold,\nRed if score is above the threshold"
            # "Select colors for user interface"
            # "Determine if score is \nabove threshold"
            # "location of python file"
            # "create json file path 2 save img score"
            # "Call python function to score img"
            # "Log Saved Image Data"
            # "Show MTN Score to user"
            # "Update Number of Images Acquired"
            # "Generate Filename"
            # "Acquire Image"
            # "Get Exposure and Gain Values"
            # "Save Image to File"
            n113 = event-data() -> ()  [unwired: 1 in, 6 out]
            n114 = local read "Saved Imaged Number"() -> (w337:i32)
            n115 = property class="Enum (strict)"(reference=w323) -> ("Value"=w324:enum16{"24.0", "15.9"})  [unwired: 1 in, 2 out]
            n116 = property class="IMAQdx"(reference=w330, "ActiveAttribute"="CameraAttributes::AcquisitionControl::ExposureTime", "ActiveAttribute"="CameraAttributes::AnalogControl::Gain") -> (reference out=w341:T6, "ValueU32"=w340:u32, "ValueU32"=w339:u32)  [unwired: 1 in, 1 out]
            n117 = call "IMAQ Cast Image 2"("Image Src"=w329, "Image Type"=w334, "error in (no error)"=w322) -> ("Image Dst Out"=w333:T1, "error out"=w332:errorcluster)  [unwired: 11 in]
            n118 = Increment(x=w337) -> (x+1=w335:i32)
            n119 = case shown="\"24.0\", Default" w324 {
              tunnel: [24.0 15.9] -> w298
              frame "24.0", Default {
              }
              frame "15.9" {
              }
            }
            n120 = property on="Image Analysis Meter" class="Slide (strict)"("DisabledEnum"=T3."Enabled" ("Disabled")) -> ()  [unwired: 2 in, 2 out]
            n121 = local write "Saved Imaged Number"(w335) -> ()
            n122 = call "Esophageal_Generate_Image_Filename.vi"("Image Number"=w335, "HRME Gain"=w339, "HRME Exposure"=w340) -> ("Notification Text"=→"Image Save Notification":string, "Image Filename"=w317:string)  [unwired: 7 in]
            n123 = local read "Representative Images"() -> (w321:path)
            n124 = Build Path(base path=w321, name or relative path=w317) -> (appended path=w346:path)
            n125 = call-poly "IMAQ Write File 2"("error in (no error)"=w332, "Image Quality"=u32 1000, "File Path"=w346, "Image"=w333) -> ("error out"=w295:errorcluster, "Image Out (duplicate)"=w344:T1)  [unwired: 6 in]
            n126 = Build Path(base path=w321, name or relative path=w317) -> (appended path=w320:path)
            n127 = local read "HRME Scores"() -> (w314:path)
            n128 = Search/Split String(string=w317, search string/char (-)=".") -> (substring before match=w315:string)  [unwired: 1 in, 2 out]
            n129 = Path To String(path=w320) -> (string=w319:string)
            n130 = Concatenate Strings(w315, ".json") -> (w313:string)
            n131 = Build Path(base path=w314, name or relative path=w313) -> (appended path=w312:path)
            n132 = Build Path(base path=path "C:/Users/EsophaHRME_Dell2/Documents/GitHub/Esophageal_HRME_Software/EsophagealDeployment/Multi_Task_Network", name or relative path="score_rep_img.py") -> (appended path=w309:path)
            n133 = Path To String(path=w312) -> (string=w306:string)
            n134 = node(w308, w309, "process_single_image", w295, "", w319, w306) -> (w307:refnum<k35>, w294:errorcluster, w299:string)  [unwired: 2 in, 2 out]
            n135 = Fract/Exp String To Number(string=w299) -> (number=w293:dbl)  [unwired: 3 in, 1 out]
            n136 = Multiply(x=w293, y=100.0) -> (x*y=w297:dbl)
            "Image Analysis Meter" <- w297
            n137 = Greater?(x=w297, y=w298) -> (0:w303:bool)
            n138 = local read "Timestamp"() -> (w326:string)
            n139 = Select(t=u32 16718848, s=w303, f=u32 65289) -> (s? t:f=w296:u32)
            n140 = local read "Log File Out"() -> (w327:refnum<file>)
            n141 = property on="Image Analysis Meter" class="Slide (strict)"(error in=w294, "Fill Color"=w296) -> (error out=w325:errorcluster)  [unwired: 1 in, 1 out]
            n142 = call "Esophageal_Datalogger_SaveButton.vi"("HRME Score"=w299, "error in (no error)"=w325, "Timestamp"=w326, "Image Name"=w317, "Log File In"=w327) -> ("error out"=w328:errorcluster)  [unwired: 5 in, 1 out]
          }
        }
        n143 = call-poly <vilib>:"DAQmx Read.vi"("task/channels in"=w119, "error in"=w105) -> ("task out"=w115:refnum<k21>, "data"=w118:bool[], "error out"=w110:errorcluster)  [unwired: 11 in]
        n144 = Index Array(array=w118, index=0) -> (element=w117:bool)
        n145 = Not(x=w117) -> (.not. x?=w116:bool)
        n146 = case shown="True" w116 {
          selector: w116 -> [w139 _]
          tunnel: w115 -> [w140 w154]
          tunnel: [w140 w153] -> w114
          tunnel: [w139 w152] -> w113
          tunnel: w110 -> [w138 w151]
          tunnel: [w138 w141] -> w104
          frame False {
          }
          frame True {
            w150 = T3."Disabled and Grayed Out" ("Disabled")
            # "Log imaging settings"
            # "Enable the pause button"
            # "Disable all controls on the front panel except the pause button"
            # "Waits until the foot pedal is done being pressed."
            n147 = while {
              tunnel: w154 -> [w162]
              tunnel: [w161] -> w153
              tunnel: [w157] -> w152
              tunnel: w151 -> [w158]
              tunnel: [w155] -> w148
              stop <- w156 stop-if-true
              n148 = call-poly <vilib>:"DAQmx Read.vi"("task/channels in"=w162, "error in"=w158) -> ("task out"=w161:refnum<k21>, "data"=w159:bool[], "error out"=w155:errorcluster)  [unwired: 11 in]
              n149 = Index Array(array=w159, index=0) -> (element=w157:bool)
              n150 = Or(x=w157, y=w155) -> (x .or. y?=w156:bool)
            }
            n151 = property on="Play Button" class="Bool"("DisabledEnum"=w150) -> ()  [unwired: 2 in, 2 out]
            n152 = property on="Calibrate" class="Bool"("DisabledEnum"=w150) -> ()  [unwired: 2 in, 2 out]
            n153 = property on="Close Program" class="Bool"("DisabledEnum"=w150) -> ()  [unwired: 2 in, 2 out]
            n154 = property on="Save Button" class="Bool"("DisabledEnum"=w150) -> ()  [unwired: 2 in, 2 out]
            n155 = property on="Pause Button" class="Bool"(error in=w148, "DisabledEnum"=T3."Enabled" ("Disabled")) -> (error out=w142:errorcluster)  [unwired: 1 in, 1 out]
            n156 = property on="HRME Exposure" class="Slide (strict)"("DisabledEnum"=w150) -> ()  [unwired: 2 in, 2 out]
            n157 = property on="HRME Gain" class="Slide (strict)"("DisabledEnum"=w150) -> ()  [unwired: 2 in, 2 out]
            n158 = property on="Auto Gain" class="Bool (strict)"("DisabledEnum"=w150) -> ()  [unwired: 2 in, 2 out]
            n159 = property on="Auto Exposure" class="Bool (strict)"("DisabledEnum"=w150) -> ()  [unwired: 2 in, 2 out]
            n160 = local read "Auto Exposure"() -> (w146:bool)
            n161 = local read "Log File Out"() -> (w147:refnum<file>)
            n162 = local read "Auto Gain"() -> (w145:bool)
            n163 = local read "HRME Exposure"() -> (w144:dbl)
            n164 = local read "HRME Gain"() -> (w143:dbl)
            n165 = call "Esophageal_Datalogger_PlayButton.vi"("Gain Value"=w143, "Auto Exposure Status"=w146, "error in (no error)"=w142, "Exposure Value"=w144, "Auto Gain Status"=w145, "Log File In"=w147) -> ("error out"=w141:errorcluster)  [unwired: 4 in, 1 out]
          }
        }
        n166 = Select(t=Esophogeal_Software_States."Imaging" ("Anal HRME States"), s=w113, f=w121) -> (s? t:f=w122:T2)
        n167 = Merge Errors(w109, w103, w104) -> (w108:errorcluster)
      }
      frame "Imaging" {
        # "Turn Red Light on to indicate frames are now being saved"
        n168 = while {
          tunnel: w366 -> [w409]
          tunnel: w365 -> [w408]
          tunnel: [w407] -> w364
          tunnel: [w388] -> w363
          tunnel: [w405] -> w352
          tunnel: w362 -> [w381]
          shift-right: [w402] -> w358
          shift-left: w361 -> [w406]
          tunnel: [w401] -> w357
          tunnel: [w399] -> w354
          tunnel: [w382] -> w353
          stop <- w400 stop-if-true
          w383 = T3."Disabled and Grayed Out" ("Disabled")
          w385 = T7 0 items=["Grayscale (U8)", "Grayscale (I16)", "Grayscale (SGL)", "Complex (CSG)", "RGB (U32)", "HSL (U32)", "RGB (U64)", "Grayscale (U16)"] ("Image Type")
          # "Converts image to array"
          # "Generate filename from timestamp"
          # "Send to producer"
          # "Read Foot Pedal Status"
          # "Acquire fastHRME Image"
          n169 = call <vilib>:"IMAQdx Grab2.vi"("error in"=w381, "Image In"=w408, "Session In"=w409) -> ("error out"=w387:errorcluster, "Image Out"=w388:T1, "Session Out"=w407:T6)  [unwired: 5 in, 1 out]
          n170 = call "IMAQ Cast Image 2"("Image Src"=w388, "Image Type"=w385, "error in (no error)"=w387) -> ("Image Dst Out"=w384:T1, "error out"=w386:errorcluster)  [unwired: 11 in]
          n171 = local write "HRME Image"(w384) -> ()
          n172 = Format Date/Time String(time format string (%c)="%H%M%S%3u") -> (date/time string=w391:string)  [unwired: 2 in]
          n173 = call "IMAQ ImageToArray"("Image"=w384) -> ("Image Pixels (U8)"=w392:u8[][])  [unwired: 3 in, 4 out]
          n174 = call-poly <vilib>:"DAQmx Read.vi"("task/channels in"=w406, "error in"=w381) -> ("task out"=w394:refnum<k21>, "data"=w396:bool[], "error out"=w393:errorcluster)  [unwired: 11 in]
          n175 = Concatenate Strings(w391, ".png" ("string")) -> (w382:string)
          n176 = call <extravilib>:"Write.vi"("element"=w382) -> ("channel"=w399:T9)  [unwired: 8 in, 2 out]
          n177 = Index Array(array=w396, index=0) -> (element=w397:bool)
          n178 = Not(x=w397) -> (.not. x?=w395:bool)
          n179 = case shown="True" w395 {
            selector: w395 -> [w411 _]
            tunnel: w394 -> [w412 w417]
            tunnel: [w412 w416] -> w402
            tunnel: [w411 w413] -> w403
            tunnel: w393 -> [w410 w415]
            tunnel: [w410 w414] -> w380
            frame False {
            }
            frame True {
              # "Waits until the foot pedal is done being pressed."
              n180 = while {
                tunnel: w417 -> [w424]
                tunnel: [w423] -> w416
                tunnel: [w420] -> w413
                tunnel: w415 -> [w419]
                tunnel: [w418] -> w414
                stop <- w420 stop-if-true
                n181 = call-poly <vilib>:"DAQmx Read.vi"("task/channels in"=w424, "error in"=w419) -> ("task out"=w423:refnum<k21>, "data"=w421:bool[], "error out"=w418:errorcluster)  [unwired: 11 in]
                n182 = Index Array(array=w421, index=0) -> (element=w420:bool)
              }
            }
          }
          n183 = property on="Save Button" class="Bool"("DisabledEnum"=w383) -> ()  [unwired: 2 in, 2 out]
          n184 = property on="Play Button" class="Bool"("DisabledEnum"=w383) -> ()  [unwired: 2 in, 2 out]
          n185 = property on="Image Analysis Meter" class="Slide (strict)"("DisabledEnum"=w383) -> ()  [unwired: 2 in, 2 out]
          n186 = Or(x="Pause Button", y=w403) -> (x .or. y?=w400:bool)
          "Pause Status" <- w400
          n187 = call <extravilib>:"Write.vi"("last element? (F)"=w400, "element"=w392) -> ("channel"=w401:T10)  [unwired: 7 in, 2 out]
          n188 = Merge Errors(w386, w380) -> (w405:errorcluster)
        }
        "Timestamp" <- w353
        n189 = call "IMAQ Create"("Image Name"="HRME Consumer") -> ("New Image"=w355:T1)  [unwired: 4 in, 1 out]
        n190 = while {
          tunnel: w357 -> [w379]
          shift-right: [w375] -> _
          shift-left: w355 -> [w371]
          tunnel: w354 -> [w374]
          stop <- w378 stop-if-true
          # "Reads image from channel, converts it into an image, then writes that image to file."
          n191 = call <extravilib>:"Read.vi"("channel"=w374) -> ("element"=w372:string)  [unwired: 6 in, 4 out]
          n192 = call <extravilib>:"Read.vi"("channel"=w379) -> ("done?"=w378:bool, "element"=w377:u8[][])  [unwired: 6 in, 3 out]
          n193 = local read "HRME Path"() -> (w369:path)
          n194 = call "IMAQ ArrayToImage"("Image Pixels (U8)"=w377, "Image"=w371) -> ("Image Out"=w376:T1)  [unwired: 8 in, 1 out]
          n195 = Build Path(base path=w369, name or relative path=w372) -> (appended path=w373:path)
          n196 = call-poly "IMAQ Write File 2"("Image Quality"=u32 1000, "File Path"=w373, "Image"=w376) -> ("Image Out (duplicate)"=w375:T1)  [unwired: 7 in, 1 out]
        }
        n197 = local read "Log File Out"() -> (w350:refnum<file>)
        n198 = call "Esophageal_Datalogger_PauseButton.vi"("error in (no error)"=w352, "Log File In"=w350) -> ("error out"=w351:errorcluster)  [unwired: 8 in, 1 out]
        "Recording" <- TRUE ("Recording")
      }
      frame "Exit" {
        # "Tell the python program to close"
        n199 = local read "Command File Location"() -> (w431:path)
        n200 = Bundle By Name(cluster=T5 {"Source"="", "Destination"="", "CMD"="newfolders", "Time"="time"} ("Output JSON File"), "CMD"="stop") -> (w434:T5)
        n201 = Flatten To JSON(anything=w434, error in (no error)=w429) -> (JSON string=w433:string, 11:w432:errorcluster)  [unwired: 1 in]
        n202 = Write to Text File(file (use dialog)=w431, text=w433, error in=w432) -> (error out=w428:errorcluster)  [unwired: 1 in, 2 out]
        n203 = local read "Log File Out"() -> (w427:refnum<file>)
        n204 = call "Esophageal_Datalogger_EndButton.vi"("error in (no error)"=w428, "Log File In"=w427) -> ("error out"=w426:errorcluster)  [unwired: 8 in, 1 out]
      }
    }
    "Anal HRME States" <- w26
    "error out" <- w17
  }
  n205 = property on="Play Button" class="Bool"("DisabledEnum"=w5) -> ()  [unwired: 2 in, 2 out]
  n206 = property on="HRME Exposure" class="Slide (strict)"("DisabledEnum"=w5) -> ()  [unwired: 2 in, 2 out]
  n207 = property on="Calibrate" class="Bool"("DisabledEnum"=w5) -> ()  [unwired: 2 in, 2 out]
  n208 = property on="HRME Gain" class="Slide (strict)"("DisabledEnum"=w5) -> ()  [unwired: 2 in, 2 out]
  n209 = property on="Close Program" class="Bool"("DisabledEnum"=w5) -> ()  [unwired: 2 in, 2 out]
  n210 = property on="Auto Gain" class="Bool (strict)"("DisabledEnum"=w5) -> ()  [unwired: 2 in, 2 out]
  n211 = property on="Save Button" class="Bool"("DisabledEnum"=w5) -> ()  [unwired: 2 in, 2 out]
  n212 = property on="Auto Exposure" class="Bool (strict)"("DisabledEnum"=w5) -> ()  [unwired: 2 in, 2 out]
  n213 = property on="Image Analysis Meter" class="Slide (strict)"("BG Color"=u32 0 ("Slider Colors:FG Color")) -> ()  [unwired: 2 in, 2 out]
  n214 = call <vilib>:"DAQmx Clear Task.vi"("task in"=w9, "error in"=w8) -> ("error out"=w2:errorcluster)  [unwired: 13 in]
  n215 = Close Python Session(session in=w1, error in=w2) -> ()  [unwired: 1 out]
